vi "exercise5_intrument.vi"() -> ()   [LabVIEW 2018]
panel:
  in  "Serial Settings:Baud Rate":u32
  out "read buffer: \nanswer from instrument":string
  out "error out":errorcluster
  in  "write buffer: \ncommand to instrument":string
  in  "VISA resource name":refnum<visa-resource-name>
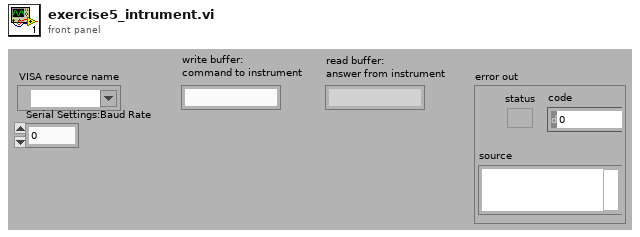
[diagram p1: front panel]
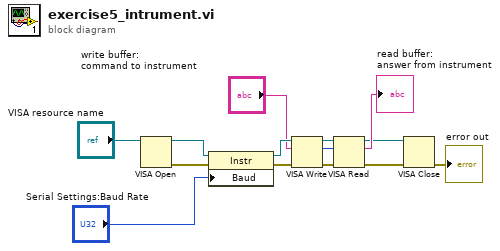
[diagram p0: block diagram]
diagram:
  n1 = VISA Open(VISA resource name="VISA resource name") -> (VISA resource name=w5:refnum<visa-resource-name>, error out=w6:errorcluster)  [unwired: 4 in]
  n2 = property class="Instr"(reference=w5, error in=w6, "Baud"="Serial Settings:Baud Rate") -> (reference out=w4:refnum<visa-resource-name>, error out=w3:errorcluster)
  n3 = VISA Write(VISA resource name=w4, write buffer="write buffer: \ncommand to instrument", error in (no error)=w3) -> (VISA resource name out=w10:refnum<visa-resource-name>, return count=w7:u32, error out=w13:errorcluster)
  n4 = VISA Read(VISA resource name=w10, byte count=w7, error in (no error)=w13) -> (VISA resource name out=w8:refnum<visa-resource-name>, read buffer=→"read buffer: \nanswer from instrument":string, error out=w12:errorcluster)  [unwired: 1 out]
  n5 = VISA Close(VISA resource name=w8, error in (no error)=w12) -> (error out=→"error out":errorcluster)
